vi "Determine Confluence Connection.vi"(8 "Error in":errorcluster caption="Error in (no error)", 11 "Confluence Settings":T1) -> (0 "Error out":errorcluster, 3 "Confluence":refnum<class "Confluence.lvclass">)   [LabVIEW 2023]
uses:
  <userlib>/_PetranWay/LabVIEW Confluence API/Source/Confluence/Confluence Connection/Confluence.lvclass
  <userlib>/_PetranWay/LabVIEW Confluence API/Source/Data Center/Confluence Data Center/Confluence Data Center.lvclass
  <userlib>/_PetranWay/LabVIEW Confluence API/Source/Cloud/Confluence Cloud/Confluence Cloud.lvclass
  <userlib>/_PetranWay/LabVIEW Confluence API/Source/Data Center/Confluence Data Center/API/Construct Confluence Data Center.vi
  <userlib>/_PetranWay/LabVIEW Confluence API/Source/Data Center/Confluence Data Center/API/Construct Confluence Data Center From Cache.vi
  <userlib>/_PetranWay/LabVIEW Confluence API/Source/Cloud/Confluence Cloud/API/Construct Confluence Cloud From Cache.vi
  <userlib>/_PetranWay/LabVIEW Confluence API/Source/Cloud/Confluence Cloud/API/Construct Confluence Cloud.vi
  <userlib>/_PetranWay/LabVIEW Atlassian API/Source/Atlassian Connection/API/Low Level/API Token Type.ctl
  <userlib>/_PetranWay/LabVIEW Atlassian API/Source/Atlassian Connection/Atlassian Connection.lvclass
  Confluence Settings.ctl
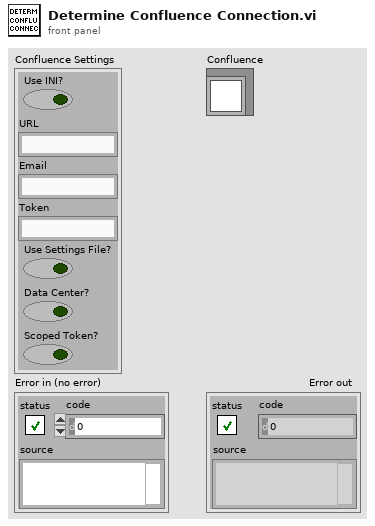
[diagram p1: front panel]
types:
  T1 = typedef "Confluence Settings.ctl" = cluster{"Use INI?":bool, "URL":string, "Email":string, "Token":string, "Use Settings File?":bool, "Data Center?":bool, "Scoped Token?":bool}
  T2 = typedef "PetranWay_Atlassian API.lvlib/Atlassian Connection.lvclass/API Token Type.ctl" = enum16{"UnScoped", "Scoped"}
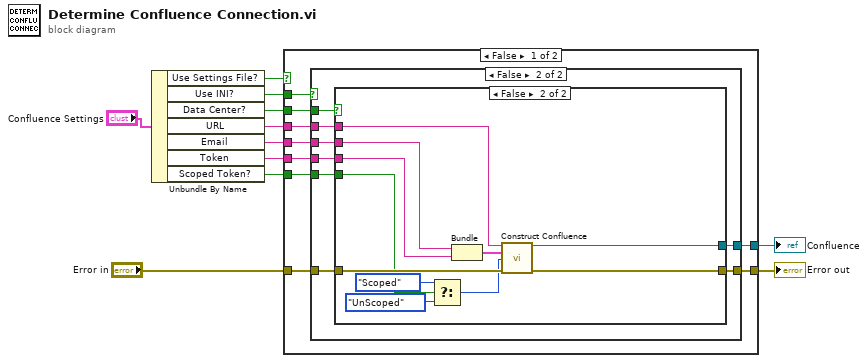
[diagram p0: block diagram]
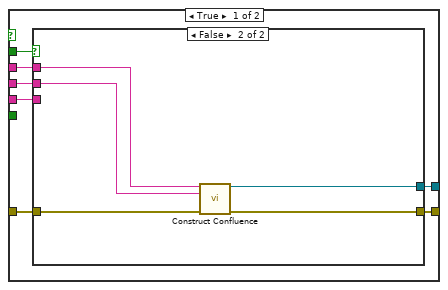
[diagram p2: hidden frame]
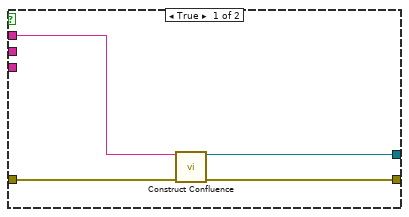
[diagram p3: hidden frame]
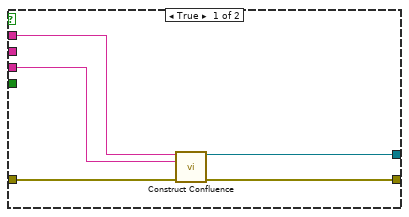
[diagram p4: hidden frame]
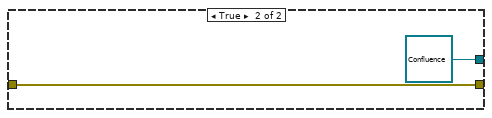
[diagram p5: hidden frame]
diagram:
  n1 = Unbundle By Name("Confluence Settings") -> ("Use Settings File?"=w10:bool, "Use INI?"=w7:bool, "Data Center?"=w6:bool, "URL"=w5:string, "Email"=w4:string, "Token"=w3:string, "Scoped Token?"=w1:bool)
  n2 = case shown="False" w10 {
    tunnel: [w14 w62] -> w9
    tunnel: "Error in" -> [w15 w62]
    tunnel: w7 -> [w20 _]
    tunnel: w6 -> [w19 _]
    tunnel: w5 -> [w18 _]
    tunnel: w4 -> [w17 _]
    tunnel: w3 -> [w16 _]
    tunnel: [w13 refnum<class "Confluence.lvclass"> refnum ("Confluence")] -> w2
    tunnel: w1 -> [w12 _]
    frame False {
      n3 = case shown="False" w20 {
        tunnel: w19 -> [w27 w44]
        tunnel: w18 -> [w26 w43]
        tunnel: w17 -> [w25 w42]
        tunnel: w16 -> [w24 w41]
        tunnel: w15 -> [w23 w40]
        tunnel: [w22 w39] -> w14
        tunnel: [w21 w38] -> w13
        tunnel: w12 -> [_ w37]
        frame True {
          n4 = case shown="False" w27 {
            tunnel: w26 -> [w28 w33]
            tunnel: w25 -> [_ w32]
            tunnel: w24 -> [_ _]
            tunnel: w23 -> [w31 w36]
            tunnel: [w30 w35] -> w22
            tunnel: [w29 w34] -> w21
            frame True {
              n5 = call-poly <userlib>:"Construct Confluence.vi"("Server URL"=w28, "error in (no error)"=w31) -> ("Confluence Data Center out"=w29:refnum<class "Confluence Data Center.lvclass">, "error out"=w30:errorcluster)  [unwired: 10 in, 2 out]
            }
            frame False {
              n6 = call-poly <userlib>:"Construct Confluence.vi"("Organization Name (https://[Organization Name].atlassian.net]"=w33, "Email Address"=w32, "error in (no error)"=w36) -> ("Confluence Cloud out"=w34:refnum<class "Confluence Cloud.lvclass">, "error out"=w35:errorcluster)  [unwired: 9 in, 2 out]
            }
          }
        }
        frame False {
          n7 = case shown="False" w44 {
            tunnel: w43 -> [w46 w57]
            tunnel: w42 -> [_ w56]
            tunnel: w41 -> [w45 w55]
            tunnel: w40 -> [w49 w60]
            tunnel: [w48 w59] -> w39
            tunnel: [w47 w58] -> w38
            tunnel: w37 -> [_ w50]
            frame True {
              n8 = call-poly <userlib>:"Construct Confluence.vi"("Your server URL"=w46, "Bearer Token"=w45, "error in (no error)"=w49) -> ("Confluence Data Center out"=w47:refnum<class "Confluence Data Center.lvclass">, "error out"=w48:errorcluster)  [unwired: 11 in]
            }
            frame False {
              n9 = Select(t=API_Token_Type."Scoped", s=w50, f=API_Token_Type."UnScoped" ("API Token Type (UnScoped)")) -> (s? t:f=w52:T2)
              n10 = Bundle("Email"=w56, "Token"=w55) -> (w54:cluster{"Email":string, "Token":string})  [unwired: 1 in]
              n11 = call-poly <userlib>:"Construct Confluence.vi"("Your Domain URL"=w57, "Email and Token"=w54, "API Token Type (UnScoped)"=w52, "error in (no error)"=w60) -> ("Confluence Cloud out"=w58:refnum<class "Confluence Cloud.lvclass">, "error out"=w59:errorcluster)  [unwired: 10 in]
            }
          }
        }
      }
    }
    frame True {
    }
  }
  "Error out" <- w9
  "Confluence" <- w2
